vi "RD_All_data(COGNEX).vi"(10 "Dara":string) -> (2 "Array":dbl[](array[numeric]))   [LabVIEW 2019]
uses:
  <vilib>/regexp/Match Regular Expression.xnode
panel:
  out "Numeric":i32
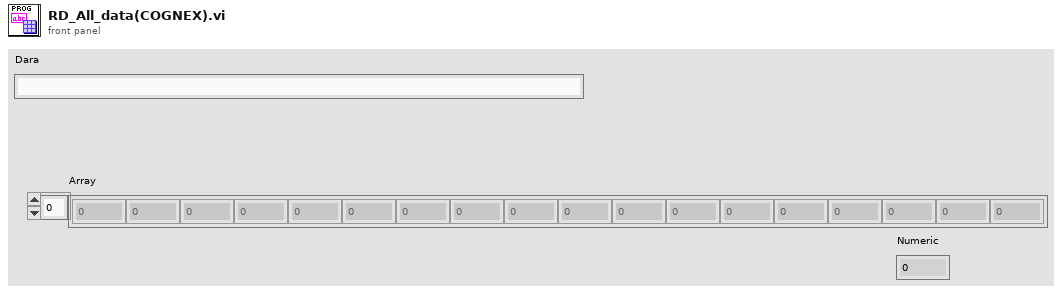
[diagram p1: front panel]
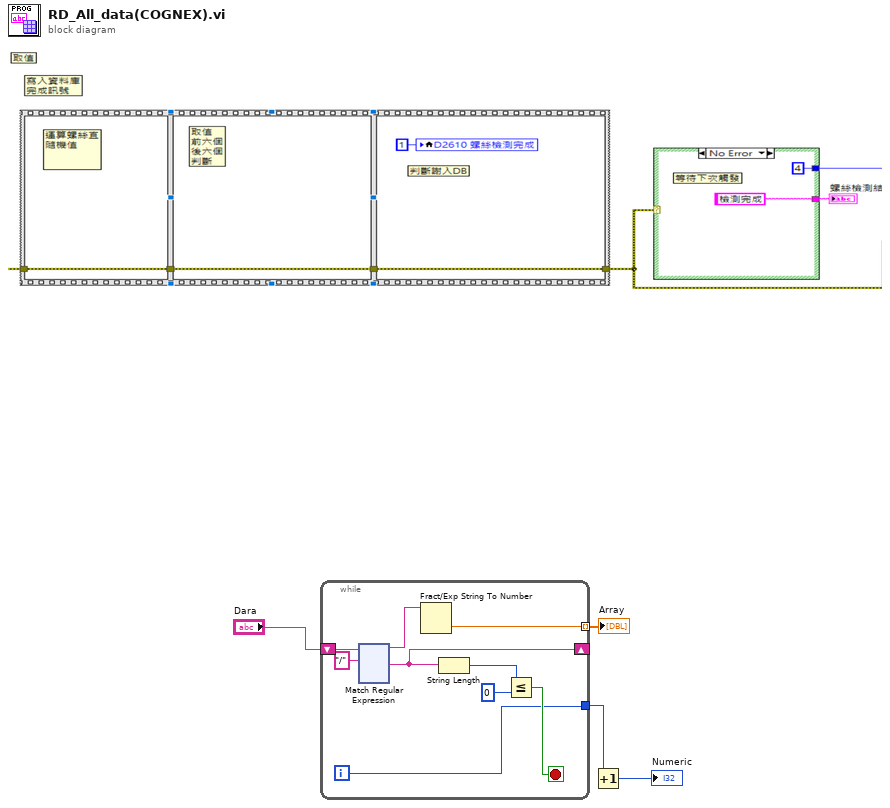
[diagram p0: block diagram]
diagram:
  n1 = while {
    shift-right: [w7] -> _
    shift-left: "Dara" -> [w12]
    tunnel: [w8] -> w3
    tunnel: [w6] -> w1 mode=indexing
    i -> [w8]
    stop <- w9 stop-if-true
    n2 = xnode "Match Regular Expression"("input string"=w12, "regular expression"="/") -> ("before match"=w11:string, "after match"=w7:string)  [unwired: 4 in, 3 out]
    n3 = Fract/Exp String To Number(string=w11) -> (number=w6:dbl)  [unwired: 3 in, 1 out]
    n4 = String Length(string=w7) -> (length=w10:i32)
    n5 = Less Or Equal?(x=w10, y=0) -> (x <= y?=w9:bool)
  }
  "Array" <- w1
  n6 = Increment(x=w3) -> (x+1=→"Numeric":i32)
